vi "configure.vi"(8 "error in (no error)":errorcluster, 9 "Path":path, 10 "Section":string, 11 "Imaq Camera in":refnum<class "Imaq Camera.lvclass">) -> (0 "error out":errorcluster, 3 "Imaq Camera out":refnum<class "Imaq Camera.lvclass">)   [LabVIEW 2022 SP3, in "Imaq Camera.lvclass"]
uses:
  Imaq Camera.lvclass
  C:/XY Stage/XY Stage/Framework/Base/Base.lvclass
  XY Stage/Framework/Base/Base.lvclass/Base.ctl
  Imaq Camera.lvclass/Imaq Camera.ctl
  XY Stage/Framework/Base/Accessors/Write Config Path.vi
  XY Stage/Framework/Base/Accessors/Write Section.vi
  <vilib>/vision/driver/NI_Vision_Acquisition_Software.lvlib
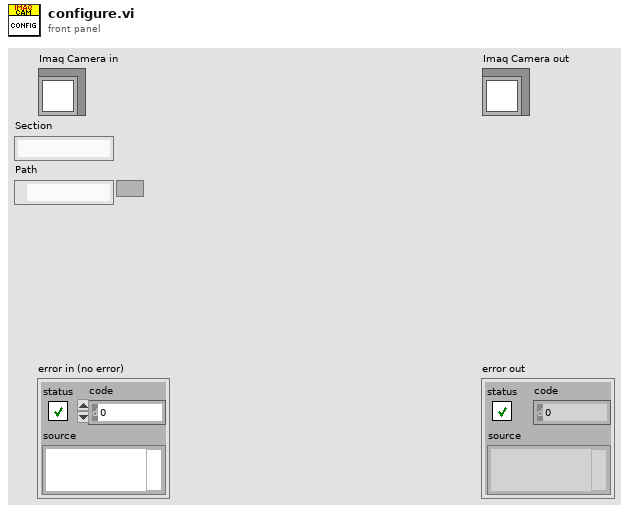
[diagram p1: front panel]
types:
  T1 = typedef "IMAQdx.ctl" = refnum<k21>
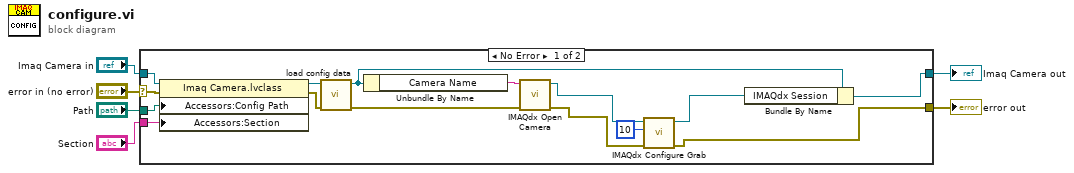
[diagram p0: block diagram]
diagram:
  n1 = case shown="No Error" "error in (no error)" {
    selector: "error in (no error)" -> [w17 w23]
    tunnel: [w8 w23] -> w5
    tunnel: [w14 w22] -> w3
    tunnel: "Imaq Camera in" -> [w21 w22]
    tunnel: "Path" -> [w20 _]
    tunnel: "Section" -> [w19 _]
    frame No Error {
      n2 = property class="Imaq Camera.lvclass"(reference=w21, error in=w17, "Accessors:Config Path"=w20, "Accessors:Section"=w19) -> (reference out=w18:refnum<class "Imaq Camera.lvclass">, error out=w16:errorcluster)
      n3 = call-dynamic "load config data.vi"("error in (no error)"=w16, "Imaq Camera in"=w18) -> ("error out"=w12:errorcluster, "Imaq Camera out"=w15:refnum<class "Imaq Camera.lvclass">)  [unwired: 8 in]
      n4 = Unbundle By Name(w15) -> ("Camera Name"=w13:string)
      n5 = call <vilib>:"IMAQdx Open Camera.vi"("error in"=w12, "Session In"=w13) -> ("error out"=w9:errorcluster, "Session Out"=w11:T1)  [unwired: 8 in]
      n6 = call <vilib>:"IMAQdx Configure Grab.vi"("error in"=w9, "Number of Buffers"=u32 10, "Session In"=w11) -> ("error out"=w8:errorcluster, "Session Out"=w10:T1)  [unwired: 7 in]
      n7 = Bundle By Name(cluster=w15, "IMAQdx Session"=w10) -> (w14:refnum<class "Imaq Camera.lvclass">)
    }
    frame Error {
    }
  }
  "error out" <- w5
  "Imaq Camera out" <- w3
